vi "Send_AddNewReference.vi"(6 "HighPriority (F)":bool, 8 "error in":errorcluster, 9 "NewRef":refnum<vi>, 11 "Queue in":refnum<queue>) -> (0 "error out":errorcluster)   [LabVIEW 2018, in "UI_Library.lvlib"]
uses:
  UI_Library.lvlib
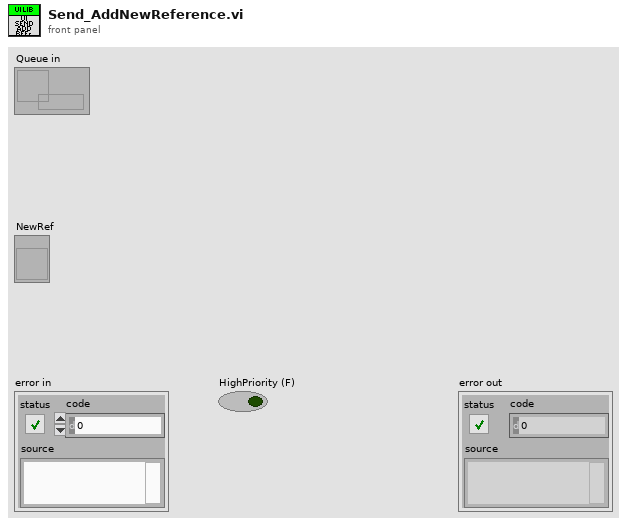
[diagram p1: front panel]
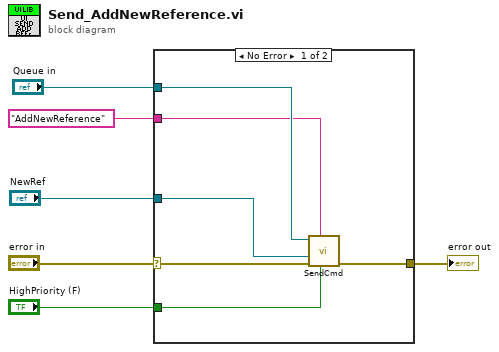
[diagram p0: block diagram]
diagram:
  n1 = case shown="No Error" "error in" {
    selector: "error in" -> [w11 w13]
    tunnel: "Queue in" -> [w12 _]
    tunnel: "NewRef" -> [w8 _]
    tunnel: "AddNewReference" ("UICmd") -> [w9 _]
    tunnel: "HighPriority (F)" -> [w7 _]
    tunnel: [w10 w13] -> w6
    frame No Error {
      n2 = call "SendCmd.vi"("HighPriority (F)"=w7, "UICmd"=w9, "error in"=w11, "Control Data"=w8, "Queue in"=w12) -> ("error out"=w10:errorcluster)  [unwired: 6 in]
    }
    frame Error {
    }
  }
  "error out" <- w6
